vi "Generate Clone Name.vi"(9 "Clone number (1)":i32=1, 11 "Fully qualified VI name":string="xyz.lvclass:abc.vi") -> (1 "Fully qualified clone name":string, 2 "Clone VI numeric suffix":string, 3 "File name of clone VI":string)   [LabVIEW 2020, in "hse-misc.lvlib"]
doc: "Given the fully qualified name of a VI (meaning the name includes any library namespace prefixes), this VI returns the name of a clone of the VI. By default, it returns the name of the first clone that gets created, but you can request the Nth clone by supplying the \"Clone number\" input.\n\nUSE WITH CAUTION. The name returned by this VI can be used with the \"Open VI Reference\" function to open a VI reference to a clone VI. This is an unsupported feature of LabVIEW (i.e. opening an additional reference to a clone VI was never intended to work but someone forgot to disable it when clones were added to LabVIEW). Opening extra references beyond the one used to create the clone (i.e. the clone's \"this VI\" reference) is known to cause instabilities, including crashes, in some situations. However, such refnums are critical for writing certain debugging tools. Be careful.\n\n____\nHAMPEL SOFTWARE ENGINEERING v3.8.0 (2023-12-18 14:41)"
uses:
  hse-misc.lvlib
panel:
  # "This VI is created by Stephen Loftus-Mercer (Aristos Queue) and available at"
  # "https://forums.ni.com/t5/Actor-Framework-Discussions/Debugging-Actors/m-p/3445827/highlight/true#M3820"
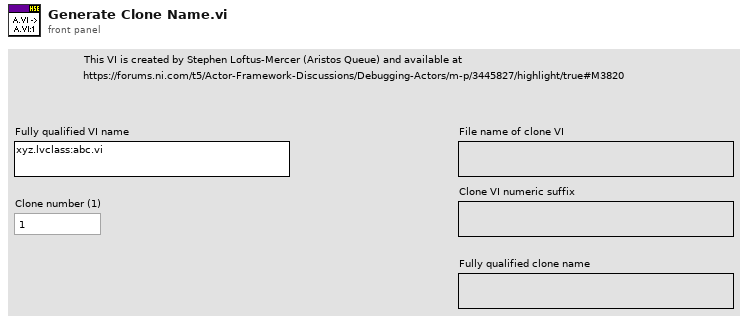
[diagram p1: front panel]
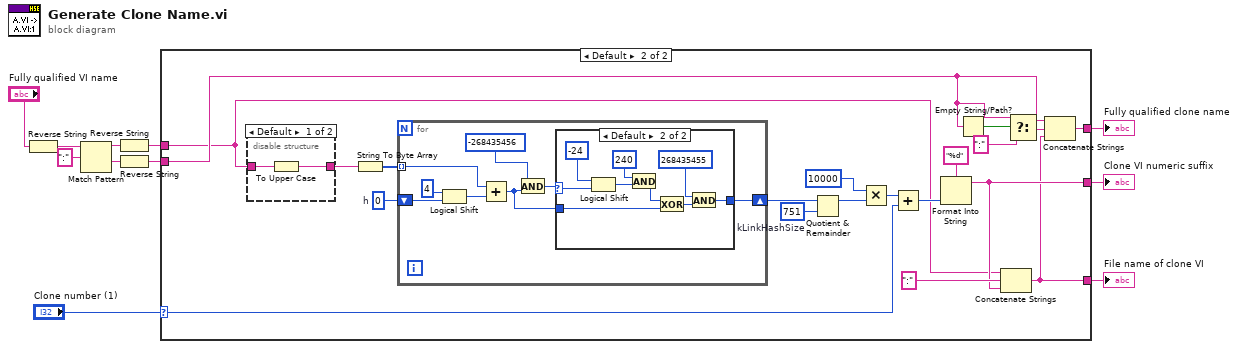
[diagram p0: block diagram]
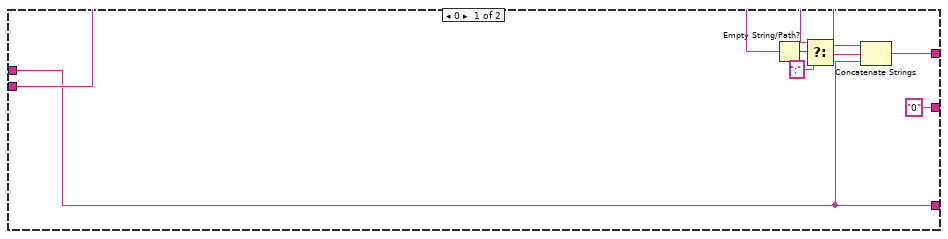
[diagram p2: hidden frame]
diagram:
  n1 = Reverse String(1:"Fully qualified VI name") -> (0:w4:string)
  n2 = Match Pattern(string=w4, regular expression=":") -> (before substring=w6:string, after substring=w7:string)  [unwired: 1 in, 2 out]
  n3 = Reverse String(1:w6) -> (0:w2:string)
  n4 = Reverse String(1:w7) -> (0:w1:string)
  n5 = case shown="Default" "Clone number (1)" {
    selector: "Clone number (1)" -> [_ w21]
    tunnel: [w12 w29] -> w11
    tunnel: ["0" w23] -> w10
    tunnel: [w13 w22] -> w9
    tunnel: w2 -> [w13 w19]
    tunnel: w1 -> [w14 w20]
    frame 0 {
      n6 = Empty String/Path?(string/path=w14) -> (empty?=w17:bool)
      n7 = Select(t=w14, s=w17, f=":") -> (s? t:f=w15:string)
      n8 = Concatenate Strings(w14, w15, w13) -> (w12:string)
    }
    frame Default {
      w34 = 751  # kLinkHashSize
      w36 = 0  # h
      n9 = disable-structure shown="Default" {
        disable-tunnel: w19 -> [w58 _]
        disable-tunnel: [w57 _] -> w38
        frame condition #0 (active) {
          n10 = To Upper Case(1:w58) -> (0:w57:string)
        }
        frame condition #1 {
        }
      }
      n11 = String To Byte Array(string=w38) -> (unsigned byte array=w37:u8[])
      n12 = for {
        tunnel: w37 -> [w43] mode=indexing
        shift-right: [w39] -> w35
        shift-left: w36 -> [w46]
        n13 = Logical Shift(y=4, x=w46) -> (x << y=w44:i32)
        n14 = Add(x=w43, y=w44) -> (x+y=w40:i32)
        n15 = And(x=-268435456, y=w40) -> (x .and. y?=w41:i32)
        n16 = case shown="Default" w41 {
          selector: w41 -> [_ w56]
          tunnel: w40 -> [w47 w51]
          tunnel: [w47 w48] -> w39
          frame 0 {
          }
          frame Default {
            n17 = Logical Shift(y=-24, x=w56) -> (x << y=w54:i32)
            n18 = And(x=240, y=w54) -> (x .and. y?=w52:i32)
            n19 = Exclusive Or(1:w51, 2:w52) -> (0:w49:i32)
            n20 = And(x=268435455, y=w49) -> (x .and. y?=w48:i32)
          }
        }
      }
      n21 = Quotient & Remainder(x=w35, y=w34) -> (x-y*floor(x/y)=w33:i32)  [unwired: 1 out]
      n22 = Multiply(x=10000, y=w33) -> (x*y=w31:i32)
      n23 = Add(x=w31, y=w21) -> (x+y=w30:i32)
      n24 = Format Into String(format string="%d", w30) -> (resulting string=w23:string)  [unwired: 2 in, 1 out]
      n25 = Empty String/Path?(string/path=w20) -> (empty?=w27:bool)
      n26 = Concatenate Strings(w19, ":" ("string"), w23) -> (w22:string)
      n27 = Select(t=w20, s=w27, f=":") -> (s? t:f=w25:string)
      n28 = Concatenate Strings(w20, w25, w22) -> (w29:string)
    }
  }
  "File name of clone VI" <- w9
  "Fully qualified clone name" <- w11
  "Clone VI numeric suffix" <- w10
